vi "Read.vi"   [LabVIEW 2014, in "T3110 & T2114.lvlib"]
uses:
  T3110 & T2114.lvlib
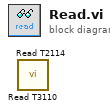
[diagram p0: block diagram]
diagram:
  n1 = call "Read T3110.vi"() -> ()  [unwired: 9 in, 3 out]
  n2 = call "Read T2114.vi"() -> ()  [unwired: 10 in, 2 out]
